vi "Tilt Platform Controller.vi"() -> ()   [LabVIEW 2014]
uses:
  <vilib>/Analysis/baseanly.llb/Mean (DBL).vi
  <vilib>/Utility/file.llb/Read From Spreadsheet File (DBL).vi
  <vilib>/Utility/file.llb/Read From Spreadsheet File (I64).vi
  <vilib>/DAQmx/create/channels.llb/DAQmx Create Channel (DO-Digital Output).vi
  <vilib>/DAQmx/create/channels.llb/DAQmx Create Channel (AI-Voltage-Basic).vi
  <vilib>/DAQmx/configure/timing.llb/DAQmx Timing (Sample Clock).vi
  <vilib>/DAQmx/configure/trigger.llb/DAQmx Start Trigger (Digital Edge).vi
  <vilib>/DAQmx/create/channels.llb/DAQmx Create Channel (AO-Voltage-Basic).vi
  <vilib>/DAQmx/write.llb/DAQmx Write (Analog DBL 1Chan 1Samp).vi
  <vilib>/DAQmx/read.llb/DAQmx Read (Analog 2D DBL NChan NSamp).vi
  <vilib>/DAQmx/write.llb/DAQmx Write (Digital 1D Bool 1Chan 1Samp).vi
  <vilib>/Utility/file.llb/Write To Spreadsheet File (DBL).vi
  <vilib>/Utility/file.llb/Write To Spreadsheet File (string).vi
  <vilib>/Analysis/NI_AALBase.lvlib
panel:
  out "Replay Loaded":bool
  out "Inclinometer":dbl
  in  "Parameter File":path
  in  "Load Sequence":bool
  in  "Replay File Path":path
  in  "Format":string="%.3f"
  in  "Delimiter":string=","
  in  "Column/Row Major":bool
  in  "Append to File?":bool=TRUE
  out "File Path":path
  out "Waveform Chart (Multiple Plots)":cluster{"mean":dbl, "mean":dbl, "mean":dbl}(graph)
  in  "Neural":bool
  in  "EMG":bool
  in  "Callib Acce":bool
  in  "Callib Load Cell":bool
  in  "Transect?":bool
  in  "Week Number":dbl
  in  "Rat ID":string
  out "4/Ev8":bool
  out "5/Ev9":bool
  out "6/Ev10":bool
  out "2/Ev6":bool
  out "1/Ev5":bool
  out "3/Ev7":bool
  in  "Baseline Angle":dbl
  out "Angle":i32
  out "Total Force (g)":i32
  out "Completed Tilts":i32
  out "Current Tilt":i32
  out "Current ITI (s)":i32
  in  "Tirgger 6":bool=TRUE
  in  "Enable Left Slow":bool=TRUE
  in  "Enable Left Medium":bool=TRUE
  in  "Enable Left Fast":bool=TRUE
  in  "Enable Right Slow":bool=TRUE
  in  "Enable Right Medium":bool=TRUE
  in  "Enable Right Fast":bool=TRUE
  out "Left Slow/Nan":i32
  out "Left Slow/8":i32
  out "Left Fast/9":i32
  out "Right Slow/6":i32
  out "Right Fast/4":i32
  out "Right Fast/Nan":i32
  out "Practice?":bool
  in  "Stop 2":bool
  in  "Pause":bool=TRUE
  in  "Tirgger 2":bool
  in  "Max Tilt Types":dbl=6.0
  in  "Total Tilts":dbl=1000.0
  in  "Reward Hold Time (s)":dbl=1.0 format="%#.6g"
  in  "Punish Hold Time (s)":dbl=1.0 format="%#.6g"
  in  "ITI Base (s)":dbl=2.0 format="%#.2g"
  in  "ITI Random Multiplier":dbl=1.0 format="%#.2g"
  in  "Clock Source":i32(slide)=1 caption="Choose a setting:" scale=0.0..1.0
  out "Reward":bool
  # "Rat Ground Reaction Forces"
  # "Clock Source"
  # "Tilt Parameters"
  # "Animal Info"
  # "Right"
  # "Left"
  # "Current Values"
  # "Enable"
  # "Enable"
  # "Callibration"
  # "File Information"
  # "Replay Sequence"
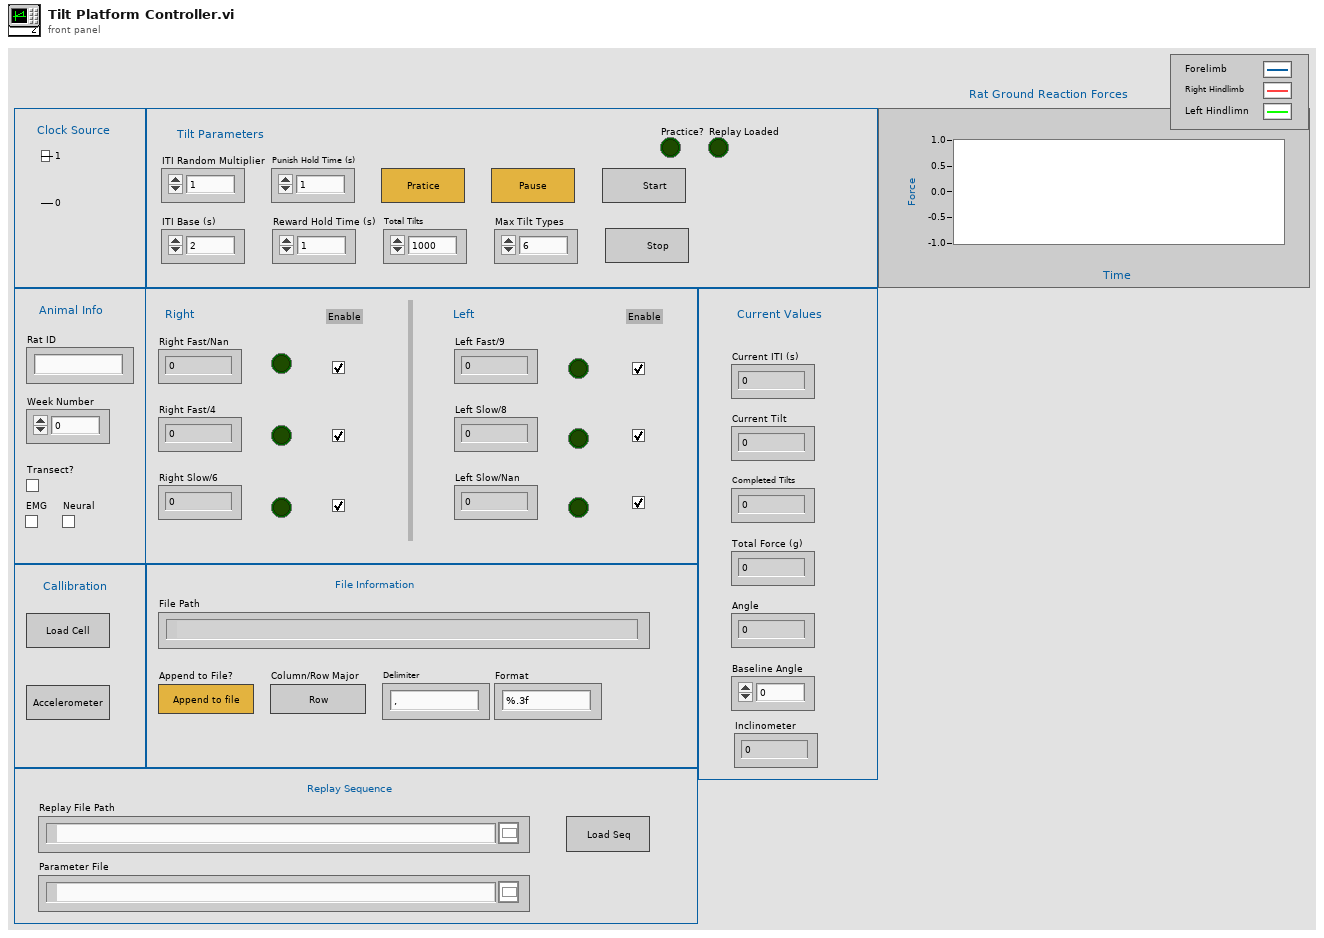
[diagram p1: front panel]
types:
  T1 = enum16{"open", "replace", "create", "open or create", "replace or create", "replace or create with confirmation"}
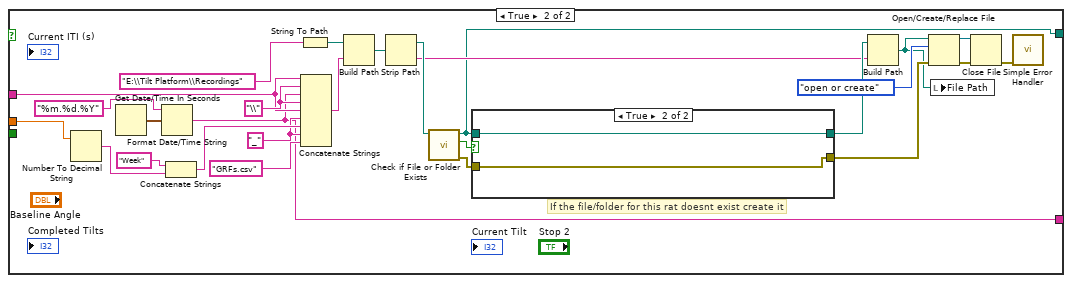
[diagram p2: hidden frame]
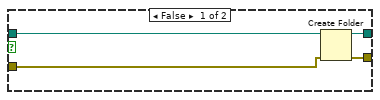
[diagram p3: hidden frame]
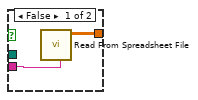
[diagram p4: hidden frame]
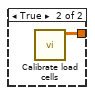
[diagram p5: hidden frame]
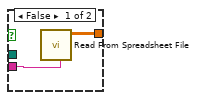
[diagram p6: hidden frame]
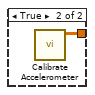
[diagram p7: hidden frame]
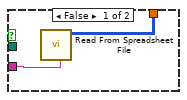
[diagram p9: hidden frame]
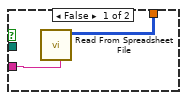
[diagram p10: hidden frame]
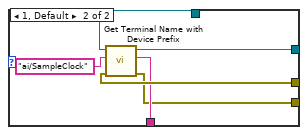
[diagram p11: hidden frame]
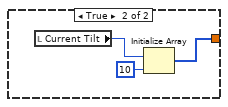
[diagram p16: hidden frame]
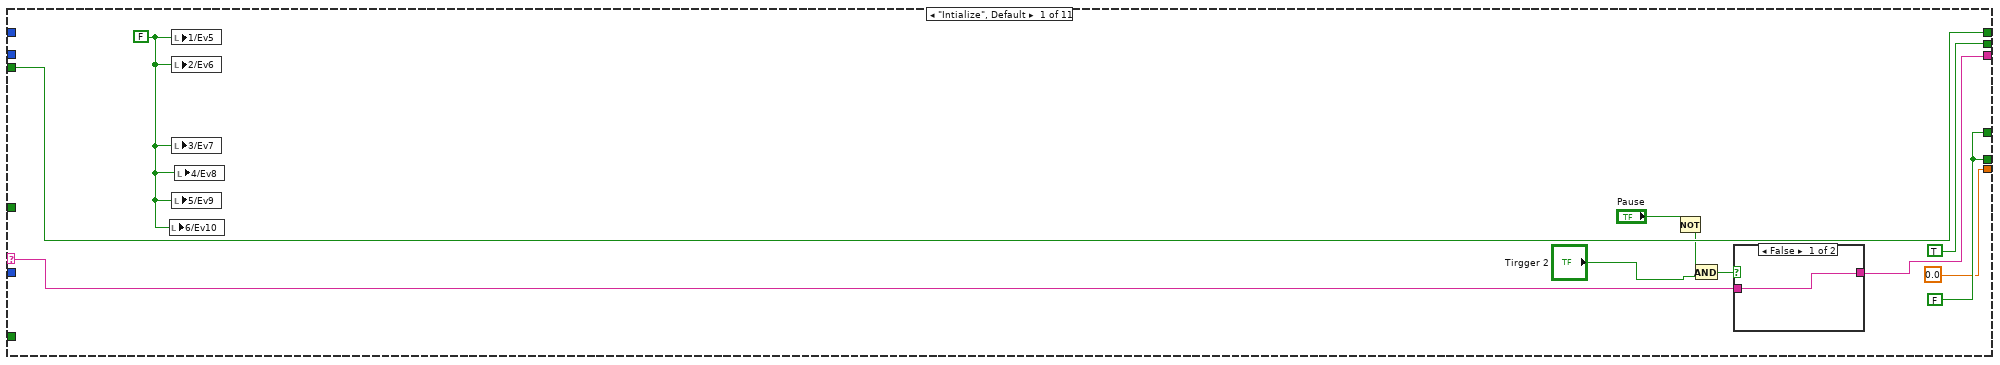
[diagram p17: hidden frame]
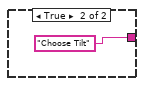
[diagram p18: hidden frame]
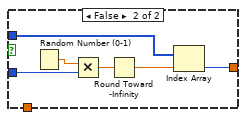
[diagram p19: hidden frame]
diagram:
  # "Turned this into a dialog\nbox -- looks nicer\nMM 2/16/2015"
  # "The GUI these items are not touched. Only through local variables"
  n1 = flat-sequence {
    tunnel: ["Tirgger 6"] -> w43
    tunnel: w43 -> [w48]
    tunnel: [w48] -> w42
    tunnel: [w51] -> w41
    tunnel: ["Transect?"] -> w24
    tunnel: [w45] -> w23
    tunnel: w42 -> [w90]
    tunnel: [w90] -> w40
    tunnel: w41 -> [w88]
    tunnel: [w89] -> w39
    tunnel: [w88] -> w38
    tunnel: [w86] -> w26
    tunnel: w24 -> [w86]
    tunnel: w23 -> [w85]
    tunnel: [w85] -> w21
    tunnel: [w107] -> w20
    tunnel: w40 -> [w106]
    tunnel: [w106] -> w18
    tunnel: w39 -> [w107]
    tunnel: [w105] -> w16
    tunnel: [w104] -> w14
    tunnel: w38 -> [w104]
    tunnel: w26 -> [w102]
    tunnel: [w102] -> w12
    tunnel: [w101] -> w10
    tunnel: w21 -> [w101]
    tunnel: w20 -> [w125]
    tunnel: [w125] -> w19
    tunnel: w18 -> [w124]
    tunnel: [w124] -> w17
    tunnel: w16 -> [w123]
    tunnel: [w123] -> w15
    tunnel: w14 -> [w122]
    tunnel: [w122] -> w13
    tunnel: w12 -> [w121]
    tunnel: [w121] -> w11
    tunnel: w10 -> [w120]
    tunnel: [w120] -> w9
    tunnel: ["Load Sequence"] -> w7
    tunnel: [w118] -> w6
    tunnel: [w202] -> w33
    tunnel: [w201] -> w34
    tunnel: w19 -> [w199]
    tunnel: [w200] -> w35
    tunnel: [w199] -> w36
    tunnel: w17 -> [w198]
    tunnel: [w198] -> w37
    tunnel: [w184] -> w32
    tunnel: [w183] -> w31
    tunnel: w15 -> [w200]
    tunnel: [w188] -> w30
    tunnel: w13 -> [w188]
    tunnel: w11 -> [w187]
    tunnel: [w187] -> w25
    tunnel: [w186] -> w22
    tunnel: w9 -> [w186]
    tunnel: [w185] -> w8
    tunnel: w7 -> [w185]
    tunnel: w6 -> [w163]
    tunnel: [w163] -> w5
    tunnel: [w169] -> w4
    tunnel: [w168] -> w3
    tunnel: w37 -> [w241]
    tunnel: w36 -> [w246]
    tunnel: w35 -> [w243]
    tunnel: w34 -> [w245]
    tunnel: w33 -> [w244]
    tunnel: w32 -> [w240]
    tunnel: w31 -> [w239]
    tunnel: [w238] -> w29
    tunnel: w30 -> [w235]
    tunnel: [w232] -> w28
    tunnel: [w231] -> w27
    tunnel: w25 -> [w229]
    tunnel: w22 -> [w228]
    tunnel: w8 -> [w227]
    tunnel: w5 -> [w226]
    tunnel: w4 -> [w225]
    tunnel: w3 -> [w224]
    tunnel: [w225] -> w2
    tunnel: [w224] -> w1
    tunnel: w29 -> [w668]
    tunnel: w28 -> [w667]
    tunnel: w27 -> [w666]
    tunnel: w2 -> [w665]
    tunnel: w1 -> [w664]
    frame #0 {
      n2 = local write "Practice?"("Tirgger 6") -> ()
    }
    frame #1 {
      n3 = Not(x=w48) -> (.not. x?=w47:bool)
      n4 = case shown="False" w47 {
        tunnel: "Transect?" -> [_ _]
        tunnel: "Week Number" -> [_ w56]
        tunnel: "Rat ID" -> [_ w55]
        tunnel: [_ w54] -> w51
        tunnel: [_ w52] -> w45
        frame False {
        }
        frame True {
          w57 = "_"
          w62 = "\\" ("string")
          # "If the file/folder for this rat doesnt exist create it"
          n5 = Number To Decimal String(number=w56) -> (decimal integer string=w77:string)  [unwired: 1 in]
          n6 = Get Date/Time In Seconds() -> (seconds since 1Jan1904=w74:timestamp)
          n7 = Format Date/Time String(time format string (%c)="%m.%d.%Y", seconds (now)=w74) -> (date/time string=w52:string)  [unwired: 1 in]
          n8 = Concatenate Strings("Week" ("string"), w77) -> (w61:string)
          n9 = String To Path(string="E:\\Tilt Platform\\Recordings") -> (path=w76:path)
          n10 = Concatenate Strings(w55, w62, w52, w62, w55, w57, w61, w57, "GRFs.csv" ("string")) -> (w59:string)
          n11 = Build Path(base path=w76, name or relative path=w59) -> (appended path=w72:path)
          n12 = Strip Path(path=w72) -> (stripped path=w71:path, name=w60:string)
          n13 = call <vilib>:"Check if File or Folder Exists.vi"("path"=w71) -> ("error out"=w69:errorcluster, "file or folder exists?"=w70:bool, "dup path"=w54:path)  [unwired: 8 in]
          n14 = case shown="True" w70 {
            tunnel: w54 -> [w82 w84]
            tunnel: w69 -> [w81 w83]
            tunnel: [w80 w84] -> w66
            tunnel: [w79 w83] -> w65
            frame False {
              n15 = Create Folder(path (use dialog)=w82, error in=w81) -> (created path=w80:path, error out=w79:errorcluster)  [unwired: 1 in, 1 out]
            }
            frame True {
            }
          }
          n16 = Build Path(base path=w66, name or relative path=w60) -> (appended path=w53:path)
          n17 = Open/Create/Replace File(file path (use dialog)=w53, error in=w65, operation (0:open)=T1."open or create") -> (refnum out=w68:refnum<file>, error out=w64:errorcluster)  [unwired: 3 in, 1 out]
          n18 = local write "File Path"(w53) -> ()
          n19 = Close File(refnum=w68, error in=w64) -> (error out=w63:errorcluster)  [unwired: 1 out]
          n20 = call <vilib>:"Simple Error Handler.vi"("error in (no error)"=w63) -> ()  [unwired: 4 in, 5 out]
        }
      }
    }
    frame #2 {
      n21 = case shown="False" "Callib Load Cell" {
        tunnel: [w92 w100] -> w89
        frame False {
          w93 = path "E:/Tilt Platform/Callibration/Load Cell/LoadCellTuningVals.csv" ("file path (dialog if empty)")
          n22 = call <vilib>:"Check if File or Folder Exists.vi"("path"=w93) -> ("file or folder exists?"=w94:bool)  [unwired: 8 in, 2 out]
          n23 = case shown="True" w94 {
            tunnel: w93 -> [_ w99]
            tunnel: [w96 w98] -> w92
            tunnel: "," ("delimiter (\\t)") -> [w95 w97]
            frame False {
              n24 = call-poly <vilib>:"Read From Spreadsheet File.vi"("delimiter (\\t)"=w95) -> ("all rows"=w96:dbl[][])  [unwired: 6 in, 4 out]
            }
            frame True {
              n25 = call-poly <vilib>:"Read From Spreadsheet File.vi"("delimiter (\\t)"=w97, "file path (dialog if empty)"=w99) -> ("all rows"=w98:dbl[][])  [unwired: 5 in, 4 out]
            }
          }
        }
        frame True {
          n26 = call "Calibrate load cells.vi"() -> ("Slope and Intercept"=w100:dbl[][])  [unwired: 11 in]
        }
      }
    }
    frame #3 {
      n27 = case shown="False" "Callib Acce" {
        tunnel: [w110 w117] -> w105
        frame False {
          w109 = path "E:/Tilt Platform/Callibration/Accelerometer/AccTuningVals.csv" ("file path (dialog if empty)")
          n28 = call <vilib>:"Check if File or Folder Exists.vi"("path"=w109) -> ("file or folder exists?"=w108:bool)  [unwired: 8 in, 2 out]
          n29 = case shown="True" w108 {
            tunnel: "," ("delimiter (\\t)") -> [w112 w116]
            tunnel: [w113 w115] -> w110
            tunnel: w109 -> [_ w114]
            frame False {
              n30 = call-poly <vilib>:"Read From Spreadsheet File.vi"("delimiter (\\t)"=w112) -> ("all rows"=w113:dbl[][])  [unwired: 6 in, 4 out]
            }
            frame True {
              n31 = call-poly <vilib>:"Read From Spreadsheet File.vi"("delimiter (\\t)"=w116, "file path (dialog if empty)"=w114) -> ("all rows"=w115:dbl[][])  [unwired: 5 in, 4 out]
            }
          }
        }
        frame True {
          n32 = call "Calibrate Accelerometer.vi"() -> ("Output"=w117:dbl[][])  [unwired: 9 in]
        }
      }
    }
    frame #4 {
      n33 = case shown="True" "Load Sequence" {
        tunnel: [_ w143] -> w118
        frame False {
        }
        frame True {
          w139 = "," ("delimiter (\\t)")
          # "Get 5th column from file"
          n34 = call <vilib>:"Check if File or Folder Exists.vi"("path"="Parameter File") -> ("file or folder exists?"=w141:bool)  [unwired: 8 in, 2 out]
          n35 = case shown="True" w141 {
            tunnel: w139 -> [w149 w152]
            tunnel: "Parameter File" -> [_ w151]
            tunnel: [w148 w150] -> w138
            frame False {
              n36 = call-poly <vilib>:"Read From Spreadsheet File.vi"("delimiter (\\t)"=w149) -> ("all rows"=w148:i64[][])  [unwired: 6 in, 4 out]
            }
            frame True {
              n37 = call-poly <vilib>:"Read From Spreadsheet File.vi"("delimiter (\\t)"=w152, "file path (dialog if empty)"=w151) -> ("all rows"=w150:dbl[][])  [unwired: 5 in, 4 out]
            }
          }
          n38 = call <vilib>:"Check if File or Folder Exists.vi"("path"="Replay File Path") -> ("file or folder exists?"=w147:bool)  [unwired: 8 in, 2 out]
          n39 = case shown="True" w147 {
            tunnel: w139 -> [w156 w159]
            tunnel: "Replay File Path" -> [_ w158]
            tunnel: [w155 w157] -> w144
            frame False {
              n40 = call-poly <vilib>:"Read From Spreadsheet File.vi"("delimiter (\\t)"=w156) -> ("all rows"=w155:i64[][])  [unwired: 6 in, 4 out]
            }
            frame True {
              n41 = call-poly <vilib>:"Read From Spreadsheet File.vi"("delimiter (\\t)"=w159, "file path (dialog if empty)"=w158) -> ("all rows"=w157:dbl[][])  [unwired: 5 in, 4 out]
            }
          }
          n42 = Index Array(array=w138, index (row)=1) -> (element=w136:dbl[])  [unwired: 1 in]
          n43 = Index Array(array=w136, index #1=0 ("index"), index #2=1 ("index"), index #3=2 ("index"), index #4=3 ("index"), index #5=4 ("index")) -> (element #1=w130:dbl, element #2=w129:dbl, element #3=w128:dbl, element #4=w127:dbl, element #5=w126:dbl)
          n44 = Index Array(array=w144, index (col)=4 ("index")) -> (element=w142:dbl[])  [unwired: 1 in]
          n45 = for {
            tunnel: [w154] -> w143 mode=indexing if=w153
            tunnel: w142 -> [w154] mode=indexing
            n46 = Not Equal To 0?(x=w154) -> (x != 0?=w153:bool)
          }
          n47 = local write "ITI Random Multiplier"(w129) -> ()
          n48 = local write "Punish Hold Time (s)"(w128) -> ()
          n49 = local write "Reward Hold Time (s)"(w127) -> ()
          n50 = local write "ITI Base (s)"(w130) -> ()
          n51 = local write "Total Tilts"(w126) -> ()
        }
      }
    }
    frame #5 {
      w189 = 10171 items=["Rising"=10280, "Falling"=10171] ("edge")
      w177 = 10123 items=["Finite Samples"=10178, "Continuous Samples"=10123, "Hardware Timed Single Point"=12522] ("sample mode")
      w192 = 10083 items=["default"=-1, "RSE"=10083, "NRSE"=10078, "Differential"=10106, "Pseudodifferential"=12529] ("input terminal configuration")
      # "Boolean logic to motor drive"
      # "Inclinometer"
      # "change back to 16"
      # "boolean for repeated sequence array"
      # "This is the repeated sequence array"
      # "ai11: inclinometer output \nai16:18 are force sensor output\nai19:21 are accelerometer output\nai22: Feedback\nai23: BMI"
      # "I am in the non-EMG case, right? - MM 2/16/2015"
      # "lines 0:2, 3-bit binary digit indicating tilt type to the arduino\nline 3, trigger for arduino to start movement"
      # "Added 'Update Signal' (line3) line to this task - MM 2/16/2015"
      # "Consolidated 3 (line0:2) outputs to arduino into one task - MM 2/16/2015"
      # "Load Cell File"
      # "Accelerometer file"
      # "Start the pin out for the tilt platform and the update trigger"
      n52 = Array Size(array=w163) -> (size(s)=w162:i32)
      n53 = Greater?(x=w162, y=0) -> (0:→"Replay Loaded":bool)
      n54 = case shown="0" "Clock Source" {
        tunnel: [_ tag "/Dev3/PFI0" ("source")] -> w191
        frame 1, Default {
        }
        frame 0 {
        }
      }
      n55 = call-poly <vilib>:"DAQmx Create Virtual Channel.vi"("maximum value"=10.0, "minimum value"=-10.0, "input terminal configuration"=w192, "physical channels"=tag "Dev3/ai4:6,Dev3/ai0:2,Dev3/ai3,Dev3/ai26,Dev3/ai27") -> ("task out"=w193:refnum<k21>, "error out"=w194:errorcluster)  [unwired: 10 in]
      n56 = call-poly <vilib>:"DAQmx Timing.vi"("task/channels in"=w193, "sample mode"=w177, "rate"=1000.0, "source"=w191, "error in"=w194) -> ("task out"=w182:refnum<k21>, "error out"=w181:errorcluster)  [unwired: 9 in]
      n57 = case shown="0" "Clock Source" {
        tunnel: w182 -> [w217 w223]
        tunnel: w181 -> [w216 w222]
        tunnel: tag "/Dev3/PFI1" ("source") -> [_ w221]
        tunnel: w189 -> [_ w220]
        tunnel: [w217 w218] -> w180
        tunnel: [w216 w219] -> w178
        frame 1, Default {
        }
        frame 0 {
          n58 = call-poly <vilib>:"DAQmx Trigger.vi"("task/channels in"=w223, "source"=w221, "edge"=w220, "error in"=w222) -> ("task out"=w218:refnum<k21>, "error out"=w219:errorcluster)  [unwired: 10 in]
        }
      }
      n59 = case shown="0" "Clock Source" {
        tunnel: w180 -> [w208 w213]
        tunnel: [w208 w212] -> w179
        tunnel: w178 -> [w207 w211]
        tunnel: [tag "/Dev3/PFI0" ("source") w210] -> _
        tunnel: [w207 w209] -> w175
        frame 0 {
        }
        frame 1, Default {
          n60 = call "Get Terminal Name with Device Prefix.vi"("error in (no error)"=w211, "Local Terminal Name"="ai/SampleClock", "task/channels in"=w213) -> ("error out"=w209:errorcluster, "Terminal Name with Device Prefix"=w210:tag, "task out"=w212:refnum<k21>)  [unwired: 6 in]
        }
      }
      n61 = call-poly <vilib>:"DAQmx Create Virtual Channel.vi"("maximum value"=5.0, "minimum value"=0.0, "physical channels"=tag "Dev3/ao0") -> ("task out"=w173:refnum<k21>, "error out"=w172:errorcluster)  [unwired: 11 in]
      n62 = call <vilib>:"DAQmx Start Task.vi"("task/channels in"=w173, "error in"=w172) -> ("task out"=w171:refnum<k21>, "error out"=w170:errorcluster)  [unwired: 12 in]
      n63 = call-poly <vilib>:"DAQmx Write.vi"("task/channels in"=w171, "data"=5.0, "error in"=w170) -> ("task out"=w169:refnum<k21>, "error out"=w168:errorcluster)  [unwired: 10 in, 1 out]
      n64 = call-poly <vilib>:"DAQmx Create Virtual Channel.vi"("lines"=tag "Dev3/port0/line0:3") -> ("task out"=w204:refnum<k21>, "error out"=w203:errorcluster)  [unwired: 13 in]
      n65 = call <vilib>:"DAQmx Start Task.vi"("task/channels in"=w179, "error in"=w175) -> ("task out"=w184:refnum<k21>, "error out"=w183:errorcluster)  [unwired: 12 in]
      n66 = call <vilib>:"DAQmx Start Task.vi"("task/channels in"=w204, "error in"=w203) -> ("task out"=w201:refnum<k21>, "error out"=w202:errorcluster)  [unwired: 12 in]
    }
    frame #6 {
      n67 = while {
        tunnel: w246 -> [w364]
        tunnel: w245 -> [w363]
        tunnel: w244 -> [w362]
        tunnel: w243 -> [w361]
        tunnel: [w360] -> w232
        tunnel: [w359] -> w231
        shift-right: [w358] -> _
        shift-left: "Intialize " -> [w330]
        tunnel: w241 -> [w357]
        tunnel: [w293] -> _
        tunnel: w240 -> [w350]
        tunnel: w239 -> [w349]
        tunnel: [w348] -> w238
        shift-right: [w342] -> _
        shift-left: FALSE ("Reset") -> [w341]
        border: TRUE -> [_]
        tunnel: w235 -> [w332]
        tunnel: [w332] -> w234
        tunnel: [w331] -> w233
        tunnel: w227 -> [w328]
        tunnel: w226 -> [w327]
        stop <- w355 stop-if-true
        (unwired) 1 ("index")
        # "remove after testing"
        # "added mean here"
        # "Consolidated 3 outputs to arduino into one task - MM 2/16/2015\n\nNOTE: Important to use 1D Bool 1Chan 1Samp (i.e. Digital -> Single Channel -> Single Sample -> 1D boolean) instance of \nwrite VI"
        # "boolean for repeated sequence array"
        # "repeated sequence array"
        # "Write one sample timestamp\nat the transitions of the feedback pin\n\nNOTE: This changes our timestamp format\nbut is the most reasonable way to work\naround the buffering problem\n\nAlso means that we need feedback pin initialized\nto true (in arduino code), to avoid a timestamp at \nfirst sample.\n\nMM 2/16/2015"
        # "Removed the TS Write? flag\nMM 2/16/2015"
        # "Send move trigger to Arduino"
        # "Changed from 10 to 1\nto avoid downsampling\nMM 2/16/2015\n\nI deleted the one. I think \nwe can let it default to -1\nJon"
        # "Feedback Pin High?"
        # "Update Digital Lines?"
        # "Can Stop?"
        # "HR"
        # "We are continiously getting data from the force sensors and the accelerometers, calculating what their voltages mean and saving the output to a file"
        n68 = local read "Total Tilts"() -> (w293:dbl)
        n69 = Not(x=w357) -> (.not. x?=w331:bool)
        n70 = call-poly <vilib>:"DAQmx Read.vi"("task/channels in"=w350, "number of samples per channel"=10, "timeout"=100.0, "error in"=w349) -> ("task out"=w348:refnum<k21>, "data"=w325:dbl[][])  [unwired: 9 in, 1 out]
        n71 = local read "Completed Tilts"() -> (w346:i32)
        n72 = Index Array(array=w325, index (row) #1=0 ("index"), index (row) #3=2 ("index"), index (row) #4=3 ("index"), index (row) #5=4 ("index"), index (row) #6=5 ("index"), index (row) #7=6 ("index (row)"), index (row) #8=7 ("index (row)"), index (row) #9=8 ("index (row)")) -> (element #1=w294:dbl[], element #2=w324:dbl[], element #3=w323:dbl[], element #4=w322:dbl[], element #5=w321:dbl[], element #6=w320:dbl[], element #7=w306:dbl[], element #8=w303:dbl[], element #9=w300:dbl[])  [unwired: 10 in]
        n73 = Greater Or Equal?(x=w346, y=w293) -> (x >= y?=w347:bool)
        n74 = Greater Or Equal?(x=w303, y=3.5) -> (x >= y?=w290:bool[])
        n75 = Or Array Elements(Boolean array=w290) -> (logical OR=w291:bool)
        n76 = Greater Or Equal?(x=w306, y=5.08) -> (x >= y?=w304:bool[])
        n77 = Or Array Elements(Boolean array=w304) -> (logical OR=w311:bool)
        n78 = local read "Completed Tilts"() -> (w344:i32)
        n79 = Subtract(x=w300, y=2.5) -> (x-y=w298:dbl[])
        n80 = local read "Baseline Angle"() -> (w337:dbl)
        n81 = local read "Current Tilt"() -> (w289:i32)
        n82 = local read "Stop 2"() -> (w339:bool)
        n83 = call "Determine Acc Angle.vi"("za"=w322, "ya"=w320, "xa"=w321, "Acc"=w361) -> ("output angle"=w295:dbl[])  [unwired: 4 in, 3 out]
        n84 = feedback-in #1(w291) -> ()
        n85 = feedback #1() -> (w333:bool)
        n86 = call "Linear Regression for Load Cell.vi"("x3"=w323, "x2"=w324, "X1"=w294, "slope-intercept"=w364) -> ("Force HL"=w352:dbl[], "Force HR"=w353:dbl[], "Force Forepaw"=w354:dbl[])  [unwired: 5 in]
        n87 = Divide(x=w298, y=0.01677) -> (x/y=w296:dbl[])
        n88 = call-poly <vilib>:"Mean.vi"("X"=w296) -> ("mean"=→"Inclinometer":dbl)  [unwired: 1 out]
        n89 = call-poly <vilib>:"Mean.vi"("X"=w295) -> ("mean"=w312:dbl)  [unwired: 1 out]
        n90 = call-poly <vilib>:"Mean.vi"("X"=w354) -> ("mean"=w315:dbl)  [unwired: 1 out]
        n91 = Or(x=w339, y=w347) -> (x .or. y?=w345:bool)
        n92 = Add(x=w337, y=w312) -> (x+y=w340:dbl)
        n93 = case shown="\"Choose Tilt\"" w330 {
          selector: w330 -> [w382 _ _ w468 w476 w487 _ _ w506 w518 w530]
          tunnel: [w381 "Tell Servo to Update" "Wait Acknowledge 1" w466 w477 w488 "Tell Servo to Return" "Wait Acknowledge 2" w505 w519 w531] -> w358
          tunnel: [w377 TRUE TRUE w464 FALSE FALSE TRUE TRUE w509 FALSE FALSE] -> w334
          tunnel: [TRUE FALSE FALSE w464 FALSE FALSE w496 FALSE w509 FALSE FALSE] -> w356
          tunnel: w289 -> [_ _ _ _ _ _ _ _ _ w516 _]
          tunnel: w344 -> [_ _ _ _ _ _ _ _ _ _ w528]
          tunnel: w341 -> [w378 w421 _ w463 _ w486 _ _ w508 _ w525]
          tunnel: [w378 w421 TRUE ("Time has Elapsed") w463 w471 w485 w496 TRUE ("Time has Elapsed") w508 w513 w529] -> w342
          tunnel: w291 -> [_ _ _ w467 w471 _ _ _ w507 w513 _]
          tunnel: w289 -> [_ _ w457 w465 w472 w480 _ _ w510 _ _]
          tunnel: [w377 FALSE TRUE w464 FALSE FALSE FALSE TRUE ("data") w509 FALSE ("data") FALSE ("data")] -> w335
          tunnel: w328 -> [_ w395 _ _ _ _ _ _ _ _ _]
          tunnel: w327 -> [_ w388 _ _ _ _ _ _ _ _ _]
          tunnel: [0.0 ("Current Tilt") w387 w457 w465 w472 w480 0.0 ("Current Tilt") 0.0 w510 0.0 ("Current Tilt") 0.0 ("Current Tilt")] -> w326
          frame "Intialize", Default {
            w377 = FALSE
            w380 = FALSE
            n94 = local write "6/Ev10"(w380) -> ()
            n95 = local write "1/Ev5"(w380) -> ()
            n96 = local write "2/Ev6"(w380) -> ()
            n97 = local write "3/Ev7"(w380) -> ()
            n98 = local write "5/Ev9"(w380) -> ()
            n99 = local write "4/Ev8"(w380) -> ()
            n100 = Not(x="Pause") -> (.not. x?=w372:bool)
            n101 = And(x=w372, y="Tirgger 2") -> (x .and. y?=w375:bool)
            n102 = case shown="False" w375 {
              tunnel: w382 -> [w383 _]
              tunnel: [w383 "Choose Tilt"] -> w381
              frame False {
              }
              frame True {
              }
            }
          }
          frame "Choose Tilt" {
            # "Multiplies the boolean value of the enable buttons time the decimal value of the tilt.\n\nIf enable is true then 1 X tilt # = tilt #  && if enable is false then 0 X tilt # = 0\n\nIt builds an array from this \n\nYou loop to remove the zeros, forming a new array\n\nIt then randomizes across this new array for whatever size 1, 2.....max tilts"
            # "Turn on an LED and increment the counter for that \nspecific tilt #"
            # "If the randomize button is chosen this will generate a psuedo-random #\nElse it will let you pick the tilt"
            n103 = Not(x=w395) -> (.not. x?=w394:bool)
            n104 = Boolean To (0,1)(Boolean=w394) -> (0, 1=w393:i16)
            n105 = local write "Reward"(FALSE ("Reward")) -> ()
            n106 = Boolean To (0,1)(Boolean="Enable Left Slow") -> (0, 1=w408:i16)
            n107 = Boolean To (0,1)(Boolean="Enable Left Medium") -> (0, 1=w407:i16)
            n108 = Boolean To (0,1)(Boolean="Enable Left Fast") -> (0, 1=w406:i16)
            n109 = Boolean To (0,1)(Boolean="Enable Right Slow") -> (0, 1=w405:i16)
            n110 = Boolean To (0,1)(Boolean="Enable Right Medium") -> (0, 1=w404:i16)
            n111 = Boolean To (0,1)(Boolean="Enable Right Fast") -> (0, 1=w403:i16)
            n112 = Multiply(x=6, y=w408) -> (x*y=w402:i32)
            n113 = Multiply(x=5, y=w407) -> (x*y=w401:i32)
            n114 = Multiply(x=4, y=w406) -> (x*y=w400:i32)
            n115 = Multiply(x=3, y=w405) -> (x*y=w399:i32)
            n116 = Multiply(x=2, y=w404) -> (x*y=w398:i32)
            n117 = Multiply(x=1, y=w403) -> (x*y=w397:i32)
            n118 = Build Array(w402, w401, w400, w399, w398, w397) -> (w392:i32[])
            n119 = Multiply(x=w392, y=w393) -> (x*y=w391:i32[])
            n120 = for {
              tunnel: [w437] -> w396 mode=indexing if=w438
              tunnel: w391 -> [w437] mode=indexing
              n121 = Not Equal To 0?(x=w437) -> (x != 0?=w438:bool)
            }
            n122 = Array Size(array=w396) -> (size(s)=w390:i32)
            n123 = Equal To 0?(x=w390) -> (x = 0?=w389:bool)
            n124 = case shown="True" w389 {
              tunnel: w396 -> [_ w434]
              tunnel: w390 -> [_ w432]
              tunnel: [w429 w431] -> w387
              tunnel: w388 -> [w430 _]
              frame True {
                n125 = local read "Completed Tilts"() -> (w426:i32)
                n126 = Multiply(x=4 ("Completed Tilts"), y=w426) -> (x*y=w427:i32)
                n127 = Index Array(array=w430, index=w427) -> (element=w429:dbl)
              }
              frame False {
                n128 = Random Number (0-1)() -> (number: 0 to 1=w436:dbl)
                n129 = Multiply(x=w436, y=w432) -> (x*y=w435:dbl)
                n130 = Round Toward -Infinity(1:w435) -> (0:w433:dbl)
                n131 = Index Array(array=w434, index=w433) -> (element=w431:i32)
              }
            }
            n132 = local write "Current Tilt"(w387) -> ()
            n133 = case shown="6" w387 {
              tunnel: TRUE -> [_ w441 w442 w445 w448 w451 w454]
              frame 0, Default {
              }
              frame 1 {
                n134 = local write "1/Ev5"(w441) -> ()
                n135 = local read "Right Fast/Nan"() -> (w439:i32)
                n136 = Increment(x=w439) -> (x+1=→"Right Fast/Nan":i32)
              }
              frame 2 {
                n137 = local write "2/Ev6"(w442) -> ()
                n138 = local read "Right Fast/4"() -> (w444:i32)
                n139 = Increment(x=w444) -> (x+1=w443:i32)
                n140 = local write "Right Fast/4"(w443) -> ()
              }
              frame 3 {
                n141 = local write "3/Ev7"(w445) -> ()
                n142 = local read "Right Slow/6"() -> (w447:i32)
                n143 = Increment(x=w447) -> (x+1=w446:i32)
                n144 = local write "Right Slow/6"(w446) -> ()
              }
              frame 4 {
                n145 = local write "6/Ev10"(w448) -> ()
                n146 = local read "Left Fast/9"() -> (w450:i32)
                n147 = Increment(x=w450) -> (x+1=w449:i32)
                n148 = local write "Left Fast/9"(w449) -> ()
              }
              frame 5 {
                n149 = local write "5/Ev9"(w451) -> ()
                n150 = local read "Left Slow/8"() -> (w453:i32)
                n151 = Increment(x=w453) -> (x+1=w452:i32)
                n152 = local write "Left Slow/8"(w452) -> ()
              }
              frame 6 {
                n153 = local write "4/Ev8"(w454) -> ()
                n154 = local read "Left Slow/Nan"() -> (w456:i32)
                n155 = Increment(x=w456) -> (x+1=w455:i32)
                n156 = local write "Left Slow/Nan"(w455) -> ()
              }
            }
          }
          frame "Tell Servo to Update" {
            # "Replaced Write VI with this boolean constant - MM 2/16/2015"
          }
          frame "Wait Acknowledge 1" {
            w464 = FALSE
            n157 = case shown="False" w467 {
              tunnel: ["Wait For Tilt To Complete" w470] -> w466
              tunnel: w468 -> [_ w470]
              frame False {
              }
              frame True {
              }
            }
          }
          frame "Wait For Tilt To Complete" {
            n158 = case shown="True" w471 {
              tunnel: [w478 "Penalty"] -> w477
              tunnel: w476 -> [w478 _]
              frame False {
              }
              frame True {
                # "Timestamp for tilt completion"
              }
            }
          }
          frame "Penalty" {
            n159 = local read "Reward"() -> (w481:bool)
            n160 = case shown="True" w481 {
              tunnel: [w490 w491] -> w484
              frame False {
                n161 = local read "Punish Hold Time (s)"() -> (w490:dbl)
              }
              frame True {
                n162 = local read "Reward Hold Time (s)"() -> (w491:dbl)
              }
            }
            n163 = call "Elapsed Time5"("Time Target (s)"=w484, "Reset"=w486) -> ("Time has Elapsed"=w485:bool)  [unwired: 10 in, 7 out]
            n164 = case shown="True" w485 {
              tunnel: [w492 "Return From Tilt"] -> w488
              tunnel: w487 -> [w492 _]
              frame False {
              }
              frame True {
              }
            }
          }
          frame "Return From Tilt" {
            w496 = FALSE
          }
          frame "Tell Servo to Return" {
          }
          frame "Wait Acknowledge 2" {
            w509 = FALSE
            n165 = case shown="True" w507 {
              tunnel: ["Wait for full return" w512] -> w505
              tunnel: w506 -> [_ w512]
              frame False {
              }
              frame True {
              }
            }
          }
          frame "Wait for full return" {
            n166 = case shown="True" w513 {
              tunnel: [w521 "Wait Inter-tilt Interval"] -> w519
              tunnel: w518 -> [w521 _]
              tunnel: w516 -> [_ _]
              frame False {
              }
              frame True {
                # "Return completion timestamp"
              }
            }
          }
          frame "Wait Inter-tilt Interval" {
            n167 = case shown="True" w525 {
              tunnel: [w534 w535] -> w526
              frame False {
                n168 = local read "Current ITI (s)"() -> (w534:i32)
              }
              frame True {
                n169 = local read "ITI Random Multiplier"() -> (w538:dbl)
                n170 = local read "ITI Base (s)"() -> (w537:dbl)
                n171 = Random Number (0-1)() -> (number: 0 to 1=w539:dbl)
                n172 = Multiply(x=w539, y=w538) -> (x*y=w536:dbl)
                n173 = Add(x=w537, y=w536) -> (x+y=w535:dbl)
                n174 = local write "Current ITI (s)"(w535) -> ()
              }
            }
            n175 = call "Elapsed Time6"("Time Target (s)"=w526, "Reset"=w525, "Auto Reset"=FALSE) -> ("Time has Elapsed"=w529:bool)  [unwired: 9 in, 7 out]
            n176 = case shown="True" w529 {
              tunnel: [w540 "Intialize"] -> w531
              tunnel: w530 -> [w540 _]
              tunnel: w528 -> [_ w543]
              frame False {
              }
              frame True {
                n177 = Increment(x=w543) -> (x+1=w542:i32)
                n178 = local write "Completed Tilts"(w542) -> ()
              }
            }
          }
        }
        n179 = call-poly <vilib>:"Mean.vi"("X"=w352) -> ("mean"=w313:dbl)  [unwired: 1 out]
        n180 = call-poly <vilib>:"Mean.vi"("X"=w353) -> ("mean"=w314:dbl)  [unwired: 1 out]
        n181 = Bundle("mean"=w315, "mean"=w314, "mean"=w313) -> (w329:cluster{"mean":dbl, "mean":dbl, "mean":dbl})  [unwired: 1 in]
        "Waveform Chart (Multiple Plots)" <- w329
        n182 = Absolute Value(x=w340) -> (abs(x)=w336:dbl)
        n183 = local write "Angle"(w336) -> ()
        n184 = Not Equal?(x=w291, y=w333) -> (x != y?=w292:bool)
        n185 = Cluster To Array(cluster=w329) -> (array=w343:dbl[])
        n186 = case shown="False" w292 {
          tunnel: [w366 w370] -> w351
          frame False {
            n187 = Initialize Array(0.0 ("Current Tilt"), 5 ("dimension size")) -> (w366:dbl[])
          }
          frame True {
            n188 = local read "Current Tilt"() -> (w369:i32)
            n189 = Initialize Array(w369, 10 ("dimension size")) -> (w370:i32[])
          }
        }
        n190 = Add Array Elements(numeric array=w343) -> (sum=w338:dbl)
        n191 = local write "Total Force (g)"(w338) -> ()
        n192 = case shown="False" w331 {
          tunnel: w354 -> [_ w648]
          tunnel: w353 -> [_ w660]
          tunnel: w352 -> [_ w659]
          tunnel: w295 -> [_ w658]
          tunnel: w351 -> [_ w650]
          tunnel: w296 -> [_ w649]
          tunnel: w290 -> [_ w647]
          tunnel: w289 -> [_ w646]
          frame False {
          }
          frame True {
            n193 = Boolean To (0,1)(Boolean=w647) -> (0, 1=w645:i16[])
            n194 = Multiply(x=w645, y=w646) -> (x*y=w644:i32[])
            n195 = Build Array(w648, w660, w659, w658, w650, w649, w644) -> (w651:dbl[][])
            n196 = local read "File Path"() -> (w657:path)
            n197 = Not(x="Column/Row Major") -> (.not. x?=w656:bool)
            n198 = call-poly <vilib>:"Write To Spreadsheet File.vi"("delimiter (\\t)"="Delimiter", "transpose? (no:F)"=w656, "format (%.3f)"="Format", "append to file? (new file:F)"="Append to File?", "2D data"=w651, "file path (dialog if empty)"=w657) -> ()  [unwired: 2 in, 1 out]
          }
        }
        n199 = case shown="True" w311 {
          frame False {
          }
          frame True {
            n200 = local write "Reward"(TRUE ("Reward")) -> ()
          }
        }
        n201 = And(x=w356, y=w345) -> (x .and. y?=w355:bool)
        n202 = case shown="True" w334 {
          tunnel: w363 -> [w545 w552]
          tunnel: w362 -> [w544 w551]
          tunnel: [w545 w550] -> w360
          tunnel: [w544 w549] -> w359
          tunnel: w335 -> [_ w548]
          tunnel: w326 -> [_ w547]
          frame False {
          }
          frame True {
            # "Send the update signal plus the correct pin combo for tilts 1-6."
            n203 = case shown="1" w547 {
              tunnel: w552 -> [w563 w578 w590 w604 w617 w630 w643]
              tunnel: w551 -> [w562 w577 w591 w603 w616 w629 w642]
              tunnel: [w555 w570 w584 w597 w610 w623 w636] -> w550
              tunnel: [w557 w574 w583 w596 w609 w622 w635] -> w549
              tunnel: w548 -> [w565 w566 w589 w602 w615 w628 w641]
              tunnel: 0.004 ("Delay Time (s)") -> [w553 w567 w579 w592 w605 w618 w631]
              frame 0, Default {
                w554 = bool[] [FALSE, FALSE, FALSE] ("data")
                n204 = Build Array (concatenate)(w554, w565) -> (w564:bool[])
                n205 = call-poly <vilib>:"DAQmx Write.vi"("task/channels in"=w563, "data"=w564, "error in"=w562) -> ("task out"=w556:refnum<k21>, "error out"=w558:errorcluster)  [unwired: 10 in, 1 out]
                n206 = call "Time Delay7"("error in (no error)"=w558, "Delay Time (s)"=w553) -> ("error out"=w559:errorcluster)  [unwired: 9 in]
                n207 = Build Array (concatenate)(w554, FALSE) -> (w560:bool[])
                n208 = call-poly <vilib>:"DAQmx Write.vi"("task/channels in"=w556, "data"=w560, "error in"=w559) -> ("task out"=w555:refnum<k21>, "error out"=w557:errorcluster)  [unwired: 10 in, 1 out]
              }
              frame 1 {
                w573 = bool[] [TRUE, FALSE, FALSE] ("data")
                n209 = Build Array (concatenate)(w573, w566) -> (w576:bool[])
                n210 = call-poly <vilib>:"DAQmx Write.vi"("task/channels in"=w578, "data"=w576, "error in"=w577) -> ("task out"=w575:refnum<k21>, "error out"=w569:errorcluster)  [unwired: 10 in, 1 out]
                n211 = call "Time Delay"("error in (no error)"=w569, "Delay Time (s)"=w567) -> ("error out"=w568:errorcluster)  [unwired: 9 in]
                n212 = Build Array (concatenate)(w573, FALSE) -> (w571:bool[])
                n213 = call-poly <vilib>:"DAQmx Write.vi"("task/channels in"=w575, "data"=w571, "error in"=w568) -> ("task out"=w570:refnum<k21>, "error out"=w574:errorcluster)  [unwired: 10 in, 1 out]
              }
              frame 2 {
                w582 = bool[] [FALSE, TRUE, FALSE] ("data")
                n214 = Build Array (concatenate)(w582, w589) -> (w588:bool[])
                n215 = call-poly <vilib>:"DAQmx Write.vi"("task/channels in"=w590, "data"=w588, "error in"=w591) -> ("task out"=w585:refnum<k21>, "error out"=w581:errorcluster)  [unwired: 10 in, 1 out]
                n216 = call "Time Delay2"("error in (no error)"=w581, "Delay Time (s)"=w579) -> ("error out"=w580:errorcluster)  [unwired: 9 in]
                n217 = Build Array (concatenate)(w582, FALSE) -> (w586:bool[])
                n218 = call-poly <vilib>:"DAQmx Write.vi"("task/channels in"=w585, "data"=w586, "error in"=w580) -> ("task out"=w584:refnum<k21>, "error out"=w583:errorcluster)  [unwired: 10 in, 1 out]
              }
              frame 3 {
                w595 = bool[] [TRUE, TRUE, FALSE] ("data")
                n219 = Build Array (concatenate)(w595, w602) -> (w601:bool[])
                n220 = call-poly <vilib>:"DAQmx Write.vi"("task/channels in"=w604, "data"=w601, "error in"=w603) -> ("task out"=w598:refnum<k21>, "error out"=w594:errorcluster)  [unwired: 10 in, 1 out]
                n221 = Build Array (concatenate)(w595, FALSE) -> (w599:bool[])
                n222 = call "Time Delay3"("error in (no error)"=w594, "Delay Time (s)"=w592) -> ("error out"=w593:errorcluster)  [unwired: 9 in]
                n223 = call-poly <vilib>:"DAQmx Write.vi"("task/channels in"=w598, "data"=w599, "error in"=w593) -> ("task out"=w597:refnum<k21>, "error out"=w596:errorcluster)  [unwired: 10 in, 1 out]
              }
              frame 4 {
                w608 = bool[] [FALSE, FALSE, TRUE] ("data")
                n224 = Build Array (concatenate)(w608, w615) -> (w614:bool[])
                n225 = call-poly <vilib>:"DAQmx Write.vi"("task/channels in"=w617, "data"=w614, "error in"=w616) -> ("task out"=w611:refnum<k21>, "error out"=w607:errorcluster)  [unwired: 10 in, 1 out]
                n226 = call "Time Delay4"("error in (no error)"=w607, "Delay Time (s)"=w605) -> ("error out"=w606:errorcluster)  [unwired: 9 in]
                n227 = Build Array (concatenate)(w608, FALSE) -> (w612:bool[])
                n228 = call-poly <vilib>:"DAQmx Write.vi"("task/channels in"=w611, "data"=w612, "error in"=w606) -> ("task out"=w610:refnum<k21>, "error out"=w609:errorcluster)  [unwired: 10 in, 1 out]
              }
              frame 5 {
                w621 = bool[] [TRUE, FALSE, TRUE] ("data")
                n229 = Build Array (concatenate)(w621, w628) -> (w627:bool[])
                n230 = call-poly <vilib>:"DAQmx Write.vi"("task/channels in"=w630, "data"=w627, "error in"=w629) -> ("task out"=w624:refnum<k21>, "error out"=w620:errorcluster)  [unwired: 10 in, 1 out]
                n231 = call "Time Delay5"("error in (no error)"=w620, "Delay Time (s)"=w618) -> ("error out"=w619:errorcluster)  [unwired: 9 in]
                n232 = Build Array (concatenate)(w621, FALSE) -> (w625:bool[])
                n233 = call-poly <vilib>:"DAQmx Write.vi"("task/channels in"=w624, "data"=w625, "error in"=w619) -> ("task out"=w623:refnum<k21>, "error out"=w622:errorcluster)  [unwired: 10 in, 1 out]
              }
              frame 6 {
                w634 = bool[] [FALSE, TRUE, TRUE] ("data")
                n234 = Build Array (concatenate)(w634, w641) -> (w640:bool[])
                n235 = call-poly <vilib>:"DAQmx Write.vi"("task/channels in"=w643, "data"=w640, "error in"=w642) -> ("task out"=w637:refnum<k21>, "error out"=w633:errorcluster)  [unwired: 10 in, 1 out]
                n236 = call "Time Delay6"("error in (no error)"=w633, "Delay Time (s)"=w631) -> ("error out"=w632:errorcluster)  [unwired: 9 in]
                n237 = Build Array (concatenate)(w634, FALSE) -> (w638:bool[])
                n238 = call-poly <vilib>:"DAQmx Write.vi"("task/channels in"=w637, "data"=w638, "error in"=w632) -> ("task out"=w636:refnum<k21>, "error out"=w635:errorcluster)  [unwired: 10 in, 1 out]
              }
            }
          }
        }
      }
      n239 = case shown="True" w233 {
        tunnel: w234 -> [_ w271]
        tunnel: "Max Tilt Types" -> [_ w262]
        tunnel: w229 -> [_ w252]
        tunnel: w228 -> [_ w248]
        frame False {
        }
        frame True {
          n240 = Boolean To (0,1)(Boolean=w252) -> (0, 1=w251:i16)
          n241 = Path To String(path=w271) -> (string=w286:string)
          n242 = Concatenate Strings(w286, "\\" ("string"), "Recording_Parameters" ("string"), "_" ("string"), w248, ".csv" ("string")) -> (w285:string)
          n243 = local read "ITI Random Multiplier"() -> (w268:dbl)
          n244 = local read "Reward Hold Time (s)"() -> (w266:dbl)
          n245 = local read "Punish Hold Time (s)"() -> (w267:dbl)
          n246 = local read "Completed Tilts"() -> (w264:i32)
          n247 = local read "Baseline Angle"() -> (w263:dbl)
          n248 = local read "ITI Base (s)"() -> (w269:dbl)
          n249 = local read "Total Tilts"() -> (w265:dbl)
          n250 = Build Array("ITI Base", "ITI Multiplier" ("element"), "Punish Hold Time" ("element"), "Reward Hold Time" ("element"), "Total Tilts" ("element"), "Complete Tilts" ("element"), "Max Tilt Type" ("element"), "Baseline Angle" ("element"), "Neural" ("element"), "EMG" ("element"), "Transect" ("element")) -> (w274:string[])
          n251 = String To Path(string=w285) -> (path=w284:path)
          n252 = Boolean To (0,1)(Boolean="Neural") -> (0, 1=w257:i16)
          n253 = Boolean To (0,1)(Boolean="EMG") -> (0, 1=w256:i16)
          n254 = Build Array(w269, w268, w267, w266, w265, w264, w262, w263, w257, w256, w251) -> (w270:dbl[])
          n255 = call-poly <vilib>:"Write To Spreadsheet File.vi"("delimiter (\\t)"="," ("delimiter (\\t)"), "1D data"=w274, "file path (dialog if empty)"=w284) -> ("new file path (Not A Path if cancelled)"=w273:path)  [unwired: 5 in]
          n256 = call-poly <vilib>:"Write To Spreadsheet File.vi"("delimiter (\\t)"="," ("delimiter (\\t)"), "append to file? (new file:F)"=TRUE, "1D data"=w270, "file path (dialog if empty)"=w273) -> ()  [unwired: 4 in, 1 out]
        }
      }
    }
    frame #7 {
      # "For Inclinometer"
      n257 = call <vilib>:"DAQmx Clear Task.vi"("task in"=w667, "error in"=w666) -> ()  [unwired: 13 in, 1 out]
      n258 = call <vilib>:"DAQmx Clear Task.vi"("task in"=w668) -> ()  [unwired: 14 in, 1 out]
      n259 = control-ref of="This VI"() -> (w671:refnum<vi>)
      n260 = call-poly <vilib>:"DAQmx Write.vi"("task/channels in"=w665, "data"=0.0, "error in"=w664) -> ("task out"=w663:refnum<k21>, "error out"=w662:errorcluster)  [unwired: 10 in, 1 out]
      n261 = invoke class="VI" method="Default Vals.Reinit All"(reference=w671) -> (reference out=w669:refnum<vi>, error out=w670:errorcluster)  [unwired: 2 in, 1 out]
      n262 = call <vilib>:"DAQmx Clear Task.vi"("task in"=w663, "error in"=w662) -> ()  [unwired: 13 in, 1 out]
      n263 = Close Reference(reference=w669, error in (no error)=w670) -> ()  [unwired: 1 out]
    }
  }
